vi "New Task from DAQmx Configuration.vi"(8 "error in":errorcluster, 11 "DAQmx Cfg":T1={"Run Mode"=0, "Sample Rate (Hz)"=51200.0, "Block Size"=5120, "Channel Table"=[], "Trigger Type"=0, "Trigger Channel"="", "Level"=0.0, "Pretrigger"=20, "Hysteresis"=0.0, "Slope"=enum."Rising"} {"Run Mode" items=["Run Once", "Continuously"]; "Block Size" min=0; "Sample Rate (Hz)" min=0.0; "Trigger Type" items=["None", "Analog Reference"]; "Channel Table"."input terminal configuration" items=["default"=-1, "RSE"=10083, "NRSE"=10078, "Differential"=10106, "Pseudodifferential"=12529]; "Channel Table"."Channel Type" items=["Voltage (V)"=0, "Charge (C)"=9, "-"=99, "SPL (Pa)"=3, "Force (lbf)"=6, "Force (N)"=1, "Acceleration (g) - IEPE"=2, "Acceleration (g) - Charge"=12, "Acceleration (g) - 4 wire DC Voltage"=22, "Velocity (in/s)"=7, "Velocity (mm/s)"=8, "Prox Probe (mil)"=4, "Prox Probe (mm)"=5]}) -> (0 "error out":errorcluster, 3 "DAQmx task":refnum<k21>)   [LabVIEW 2024, in "Dynamic Signal Acquisition (Interactive) UI.lvlib"]
doc: "Maps DAQmx configuration to separate configuration for channels, trigger, and timing, and then calls subVI to create and configure DAQmx task."
uses:
  SFPDAQ Configuration.ctl
  SFPDAQmx Channel Info.ctl
  <vilib>/addons/_NISVFA/_Shared subVIs/Controls/svc_Analog Level Trigger Configuration.ctl
  <vilib>/addons/Sound and Vibration/svt_DAQmx/subVIs/Run Mode.ctl
  Dynamic Signal Acquisition (Interactive) UI.lvlib
  <vilib>/addons/Sound and Vibration/svt_DAQmx/subVIs/SV_DAQmx.lvlib
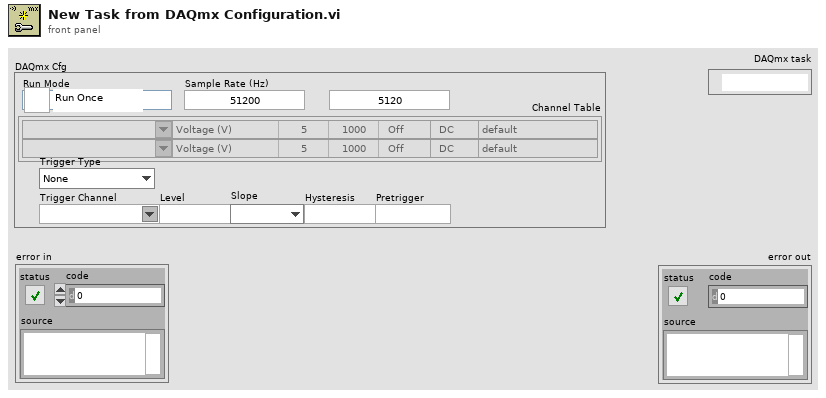
[diagram p1: front panel]
types:
  T1 = typedef "Dynamic Signal Acquisition (Interactive) UI.lvlib/SFPDAQ Configuration.ctl" = cluster{"Run Mode":u16, "Sample Rate (Hz)":dbl, "Block Size":i32, "Channel Table":T2[], "Trigger Type":u16, "Trigger Channel":string, "Level":dbl, "Pretrigger":i32, "Hysteresis":dbl, "Slope":enum16{"Falling", "Rising"}}
  T2 = typedef "Dynamic Signal Acquisition (Interactive) UI.lvlib/SFPDAQmx Channel Info.ctl" = cluster{"DAQmx Channel":tag, "Channel Type":u16, "Max":dbl, "Sensitivity":dbl, "Coupling":enum16{"AC", "DC"}, "input terminal configuration":i32, "excitation":enum16{"Off", "Min", "Max"}}
  T3 = typedef "svc_Analog Level Trigger Configuration.ctl" = cluster{"level":dbl, "slope":u16, "hysteresis":dbl}
  T4 = cluster{"enable":bool, "channel":string, "level trigger configuration":T3, "pretrigger":i32}
  T5 = typedef "SV_DAQmx.lvlib/Run Mode.ctl" = u16
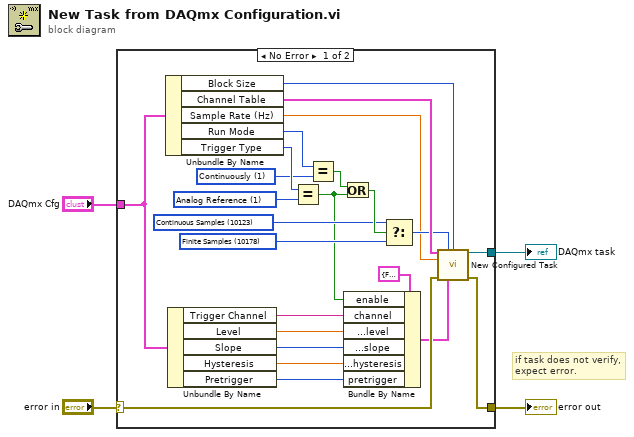
[diagram p0: block diagram]
diagram:
  # "if task does not verify,\nexpect error."
  n1 = case shown="No Error" "error in" {
    selector: "error in" -> [w6 w29]
    tunnel: [w28 _] -> w4
    tunnel: "DAQmx Cfg" -> [w8 _]
    tunnel: [w14 w29] -> w1
    frame No Error {
      w22 = T5 1 items=["Once", "Continuously"] ("Run Mode")
      w18 = 10178 items=["Finite Samples"=10178, "Continuous Samples"=10123, "Hardware Timed Single Point"=12522] ("sample mode")
      w19 = 10123 items=["Finite Samples"=10178, "Continuous Samples"=10123, "Hardware Timed Single Point"=12522] ("sample mode")
      w25 = u16 1 items=["None", "Analog Reference"] ("Trigger Type")
      n2 = Unbundle By Name(w8) -> ("Block Size"=w16:i32, "Channel Table"=w21:T2[], "Sample Rate (Hz)"=w15:dbl, "Run Mode"=w20:u16, "Trigger Type"=w26:u16)
      n3 = Unbundle By Name(w8) -> ("Trigger Channel"=w13:string, "Level"=w12:dbl, "Slope"=w11:enum16{"Falling", "Rising"}, "Hysteresis"=w10:dbl, "Pretrigger"=w9:i32)
      n4 = Equal?(x=w26, y=w25) -> (x = y?=w7:bool)
      n5 = Equal?(x=w20, y=w22) -> (x = y?=w24:bool)
      n6 = Or(x=w24, y=w7) -> (x .or. y?=w23:bool)
      n7 = Bundle By Name(cluster=T4 {"enable"=FALSE, "channel"="", "level trigger configuration"={"level"=0.0, "slope"=0, "hysteresis"=0.0}, "pretrigger"=0} ("analog reference trigger configuration"), "enable"=w7, "channel"=w13, "level trigger configuration.level"=w12, "level trigger configuration.slope"=w11, "level trigger configuration.hysteresis"=w10, "pretrigger"=w9) -> (w5:T4)
      n8 = Select(t=w19, s=w23, f=w18) -> (s? t:f=w17:i32)
      n9 = call "New Configured Task.vi"("channel table"=w21, "sample mode"=w17, "block size"=w16, "sample rate"=w15, "error in"=w6, "analog reference trigger configuration"=w5) -> ("DAQmx analog input task"=w28:refnum<k21>, "error out"=w14:errorcluster)  [unwired: 7 in, 1 out]
    }
    frame Error {
    }
  }
  "DAQmx task" <- w4
  "error out" <- w1
